vi "Element Init.vi"(7 "VolatusAPI":refnum<class "VolatusAPI.lvclass">, 8 "error in (no error)":errorcluster, 10 "JSON":string, 11 "LoggingControl in":refnum<class "LoggingControl.lvclass">) -> (0 "error out":errorcluster, 3 "LoggingControl out":refnum<class "LoggingControl.lvclass">)   [LabVIEW 2020, in "VolatusGUIElements.lvlib" / "LoggingControl.lvclass"]
uses:
  LoggingControl.lvclass
  C:/dev/lv20CE/relink/lv-volatus/VolatusGUI/GUI Element/GUI Element.lvclass
  Volatus/VolatusAPI/VolatusAPI.lvclass
  JSON.ctl
  Prompt Result.ctl
  Prompt Action.ctl
  LoggingControl.lvclass/LoggingControl.ctl
  VolatusGUI/GUI Element/GUI Element.lvclass/GUI Element.ctl
  6b4406ff-dbb0-478f-9794-4f2464f74e8d.vi
  <vilib>/JDP Science/JSONtext/JSON text to Variant.vi
  <vilib>/JDP Science/JSONtext/LVClass Serializer/JSONtext LVClass Serializer.lvclass
  VolatusGUI/GUI Element/GUI Element.lvclass
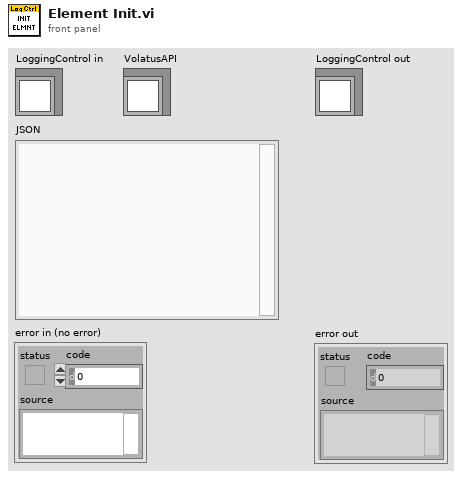
[diagram p1: front panel]
types:
  T1 = typedef "VolatusGUIElements.lvlib/LoggingControl.lvclass/Prompt Result.ctl" = cluster{"Action":T2, "Series":string, "Timestamp":string}
  T2 = typedef "VolatusGUIElements.lvlib/LoggingControl.lvclass/Prompt Action.ctl" = enum16{"Cancelled", "Started"}
  T3 = typedef "VolatusGUIElements.lvlib/LoggingControl.lvclass/JSON.ctl" = cluster{"Targets":string[]}
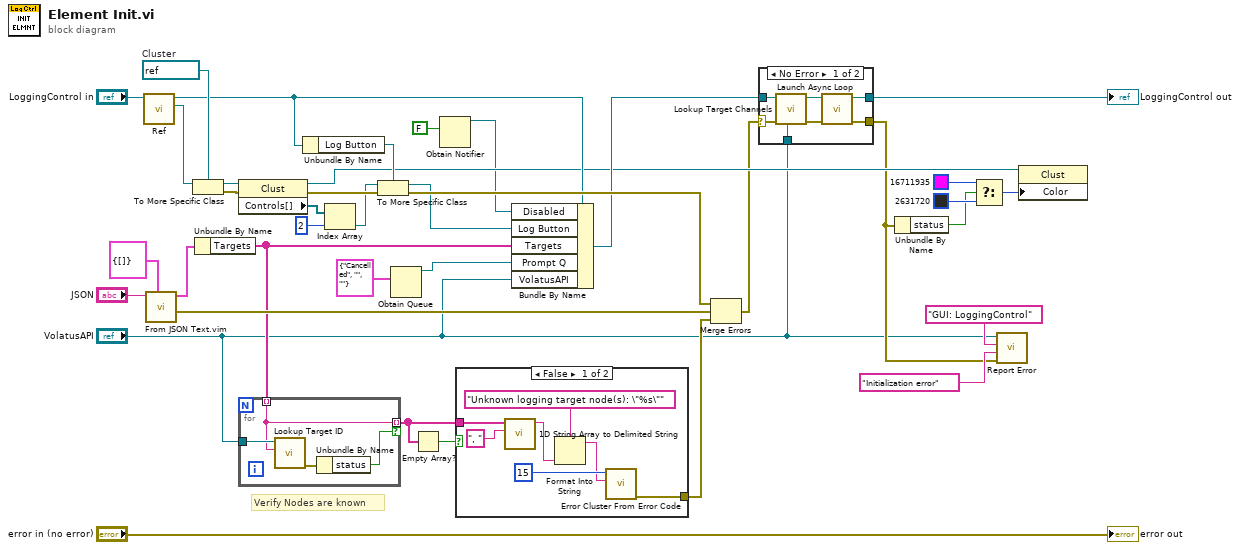
[diagram p0: block diagram]
diagram:
  w34 = refnum<vi> refnum  # Cluster
  # "Verify Nodes are known"
  n1 = call "Ref.vi"("GUI Element in"="LoggingControl in") -> ("Ref"=w35:refnum<vi>, "GUI Element out"=w28:refnum<class "LoggingControl.lvclass">)  [unwired: 9 in]
  n2 = call "From JSON Text.vim"("Data Type and Default Value"=T3 {"Targets"=[]} ("JSON"), "JSON"="JSON") -> ("error out"=w21:errorcluster, "Data out"=w22:T3)  [unwired: 8 in]
  n3 = To More Specific Class(target class=w34, reference=w35) -> (specific class reference=w33:refnum<vi>, error out=w32:errorcluster)  [unwired: 1 in]
  n4 = Unbundle By Name(w22) -> ("Targets"=w20:string[])
  n5 = property class="Clust"(reference=w33, error in=w32) -> (reference out=w15:refnum<vi>, error out=w37:errorcluster, "Controls[]"=w31:refnum<vi>[])
  n6 = for {
    tunnel: "VolatusAPI" -> [w42]
    tunnel: w20 -> [w40] mode=indexing
    tunnel: [w40] -> w18 mode=indexing if=w39
    n7 = call "Lookup Target ID.vi"("Target Name"=w40, "VolatusAPI in"=w42) -> ("error out"=w41:errorcluster)  [unwired: 6 in, 3 out]
    n8 = Unbundle By Name(w41) -> ("status"=w39:bool)
  }
  n9 = Unbundle By Name(w28) -> ("Log Button"=w27:refnum<vi>)
  n10 = Index Array(array=w31, index=2) -> (element=w29:refnum<vi>)
  n11 = To More Specific Class(target class=w27, reference=w29, error in=w37) -> (specific class reference=w25:refnum<vi>, error out=w38:errorcluster)
  n12 = Obtain Queue(element data type=T1 {"Action"=enum."Cancelled", "Series"="", "Timestamp"=""} ("Prompt Result")) -> (queue out=w4:refnum<queue>)  [unwired: 4 in, 2 out]
  n13 = Empty Array?(array=w18) -> (empty?=w19:bool)
  n14 = Obtain Notifier(notification data type=FALSE) -> (notifier out=w1:refnum<notifier>)  [unwired: 3 in, 2 out]
  n15 = case shown="False" w19 {
    tunnel: w18 -> [w49 _]
    tunnel: [w43 _] -> w17
    frame False {
      n16 = call <vilib>:"1D String Array to Delimited String.vi"("delimiter"=", ", "string array"=w49) -> ("delimited string"=w46:string)  [unwired: 9 in]
      n17 = Format Into String(format string="Unknown logging target node(s): \"%s\"", w46) -> (resulting string=w44:string)  [unwired: 2 in, 1 out]
      n18 = call <vilib>:"Error Cluster From Error Code.vi"("error message (\"\")"=w44, "error code (0)"=15) -> ("error out"=w43:errorcluster)  [unwired: 7 in]
    }
    frame True {
    }
  }
  n19 = Bundle By Name(cluster=w28, "Disabled"=w1, "Log Button"=w25, "Targets"=w20, "Prompt Q"=w4, "VolatusAPI"="VolatusAPI") -> (w26:refnum<class "LoggingControl.lvclass">)
  n20 = Merge Errors(w38, w21, w17) -> (w7:errorcluster)
  n21 = case shown="No Error" w7 {
    selector: w7 -> [w55 w58]
    tunnel: w26 -> [w56 w57]
    tunnel: [w50 w57] -> w8
    tunnel: [w52 w58] -> w6
    tunnel: "VolatusAPI" -> [w53 _]
    frame No Error {
      n22 = call "Lookup Target Channels.vi"("VolatusAPI"=w53, "error in (no error)"=w55, "LoggingControl in"=w56) -> ("error out"=w54:errorcluster, "LoggingControl out"=w51:refnum<class "LoggingControl.lvclass">)  [unwired: 7 in]
      n23 = call "Launch Async Loop.vi"("error in (no error)"=w54, "LoggingControl in"=w51) -> ("error out"=w52:errorcluster, "LoggingControl out"=w50:refnum<class "LoggingControl.lvclass">)  [unwired: 8 in]
    }
    frame Error {
    }
  }
  "LoggingControl out" <- w8
  n24 = Unbundle By Name(w6) -> ("status"=w10:bool)
  n25 = Select(t=u32 16711935 ("Color"), s=w10, f=u32 2631720 ("Color")) -> (s? t:f=w12:u32)
  n26 = call "Report Error.vi"("error in (no error)"=w6, "Message"="Initialization error", "Context"="GUI: LoggingControl", "VolatusAPI in"="VolatusAPI") -> ()  [unwired: 6 in, 2 out]
  n27 = property class="Clust"(reference=w15, "Color"=w12) -> ()  [unwired: 1 in, 2 out]
  "error out" <- "error in (no error)"
